vi "Igor_SaveWavesToFile.vi"(8 "error in (no error)":errorcluster, 9 "Wavenames":string[](array[string])=["Wave1", "Wave2", "Wave3"], 10 "Path":path=path "C:/Users/Albro/Desktop/A New File3.txt", 11 "Application In":refnum<k7>) -> (0 "error out":errorcluster, 3 "Application Out":refnum<k7>)   [LabVIEW 2020]
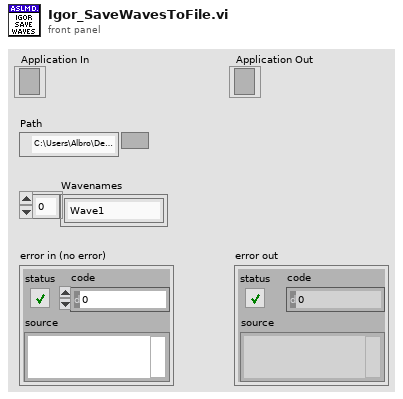
[diagram p1: front panel]
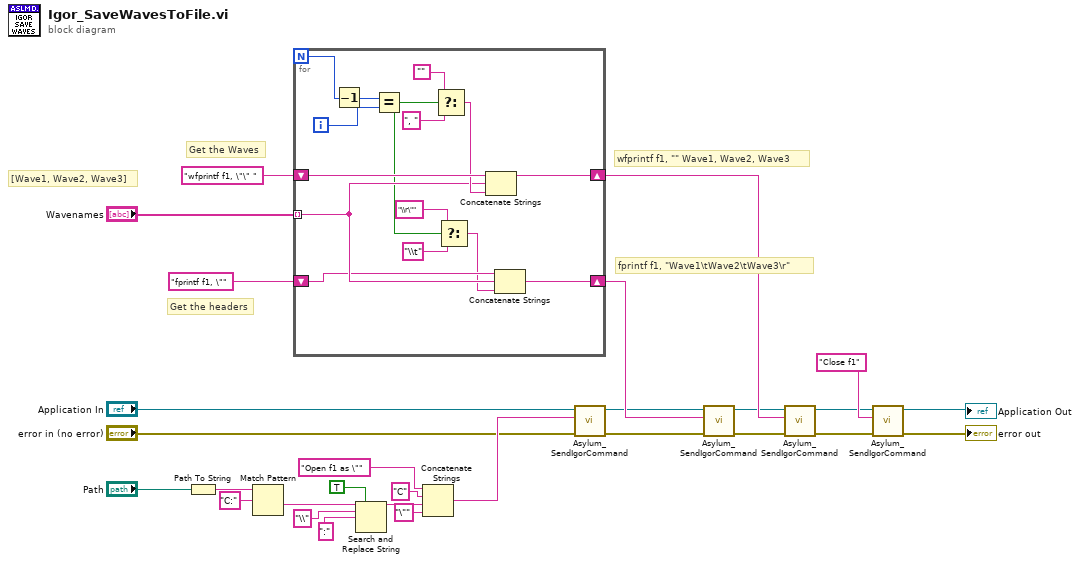
[diagram p0: block diagram]
diagram:
  # "[Wave1, Wave2, Wave3]"
  # "wfprintf f1, \"\" Wave1, Wave2, Wave3"
  # "fprintf f1, \"Wave1\\tWave2\\tWave3\\r\""
  # "Get the Waves"
  # "Get the headers"
  n1 = Path To String(path="Path") -> (string=w9:string)
  n2 = Match Pattern(string=w9, regular expression="C:") -> (after substring=w13:string)  [unwired: 1 in, 3 out]
  n3 = for {
    N -> [w41]
    tunnel: "Wavenames" -> [w34] mode=indexing
    shift-right: [w42] -> w24
    shift-left: "wfprintf f1, \"\" " -> [w43]
    shift-right: [w32] -> w25
    shift-left: "fprintf f1, \"" -> [w33]
    i -> [w39]
    n4 = Decrement(x=w41) -> (x-1=w40:i32)
    n5 = Equal?(x=w40, y=w39) -> (x = y?=w30:bool)
    n6 = Select(t="", s=w30, f=", ") -> (s? t:f=w37:string)
    n7 = Select(t="\\r\"" ("f"), s=w30, f="\\t") -> (s? t:f=w29:string)
    n8 = Concatenate Strings(w43, w34, w37) -> (w42:string)
    n9 = Concatenate Strings(w33, w34, w29) -> (w32:string)
  }
  n10 = Search and Replace String(replace all?=TRUE ("replace all? (F)"), input string=w13, search string="\\", replace string=":" ("replace string (\"\")")) -> (result string=w11:string)  [unwired: 4 in, 3 out]
  n11 = Concatenate Strings("Open f1 as \"" ("command"), "C" ("string"), w11, "\"" ("string")) -> (w3:string)
  n12 = call <vilib>:"Asylum_SendIgorCommand.vi"("error in (no error)"="error in (no error)", "command"=w3, "Application In"="Application In") -> ("error out"=w16:errorcluster, "Application Out"=w15:refnum<k7>)  [unwired: 5 in, 2 out]
  n13 = call <vilib>:"Asylum_SendIgorCommand.vi"("error in (no error)"=w16, "command"=w25, "Application In"=w15) -> ("error out"=w22:errorcluster, "Application Out"=w18:refnum<k7>)  [unwired: 5 in, 2 out]
  n14 = call <vilib>:"Asylum_SendIgorCommand.vi"("error in (no error)"=w22, "command"=w24, "Application In"=w18) -> ("error out"=w21:errorcluster, "Application Out"=w17:refnum<k7>)  [unwired: 5 in, 2 out]
  n15 = call <vilib>:"Asylum_SendIgorCommand.vi"("error in (no error)"=w21, "command"="Close f1", "Application In"=w17) -> ("error out"=→"error out":errorcluster, "Application Out"=→"Application Out":refnum<k7>)  [unwired: 5 in, 2 out]
